vi "Acquisition Message Loop.vi"(8 "error in (no error)":errorcluster, 9 "Data Queue":refnum<queue>, 10 "Data Notifier":refnum<notifier>, 11 "Message Queues":T1) -> (0 "error out":errorcluster)   [LabVIEW 2016, in "Acquisition.lvlib"]
doc: "Message loop for handling messages pertaining to the acquisition of data from the hardware."
uses:
  Acquisition.lvlib
  support/Message Queue/All Message Queues.ctl
  support/Message Queue/Message Cluster.ctl
  Acquisition State.ctl
  Settings/Settings.ctl
  Logging/Logging Configuration.ctl
  Hardware Configuration.ctl
  support/Message Queue/Enqueue Message (Single).vi
  <vilib>/Utility/error.llb/Error Cluster From Error Code.vi
  <vilib>/ErrorRing/Error Ring.xnode
  support/Message Queue/Message Queue.lvlib
  Logging/Logging.lvlib
  Settings/Settings.lvlib
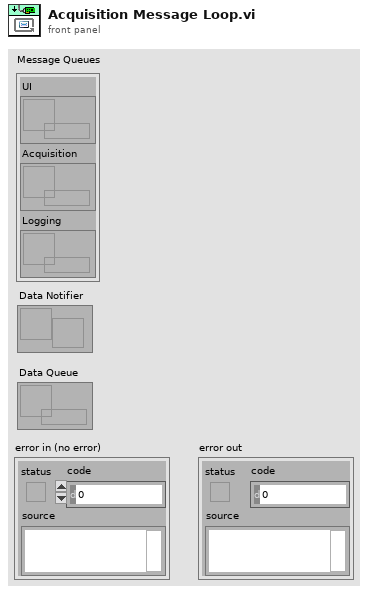
[diagram p1: front panel]
types:
  T1 = typedef "Message Queue.lvlib/All Message Queues.ctl" = cluster{"UI":refnum<queue>, "Acquisition":refnum<queue>, "Logging":refnum<queue>}
  T2 = typedef "Acquisition.lvlib/Acquisition State.ctl" = enum16{"Idle", "Acquiring"}
  T3 = typedef "Settings.lvlib/Settings.ctl" = cluster{"Logging Configuration":T4, "Hardware Config":cluster{"Bautrate":string, "VISA":T5}, "Advance Setting":cluster{"PWM_Step":dbl, "PWM_MIN":dbl, "PWM_MAX":dbl, "DeadZone(mv)":dbl, "SamCycle(ms)":dbl, "Bang-BangTerm":dbl, "ecS":dbl, "ecM":dbl, "ecL":dbl, "eS":dbl, "eM":dbl, "eL":dbl, "Kd F":dbl, "Ki F":dbl, "Kp F":dbl, "Kd":dbl, "Ki":dbl, "Kp":dbl}, "FuzzyMap":cluster{"Table":string[][]}, "ControlMode":cluster{"Control":enum32{"1", "2", "4"}}}
  T4 = typedef "Logging.lvlib/Logging Configuration.ctl" = cluster{"Log File Base Path":path, "save file":bool, "refnum out":refnum<file>}
  T5 = typedef "Acquisition.lvlib/Hardware Configuration.ctl" = refnum<visa-resource-name>
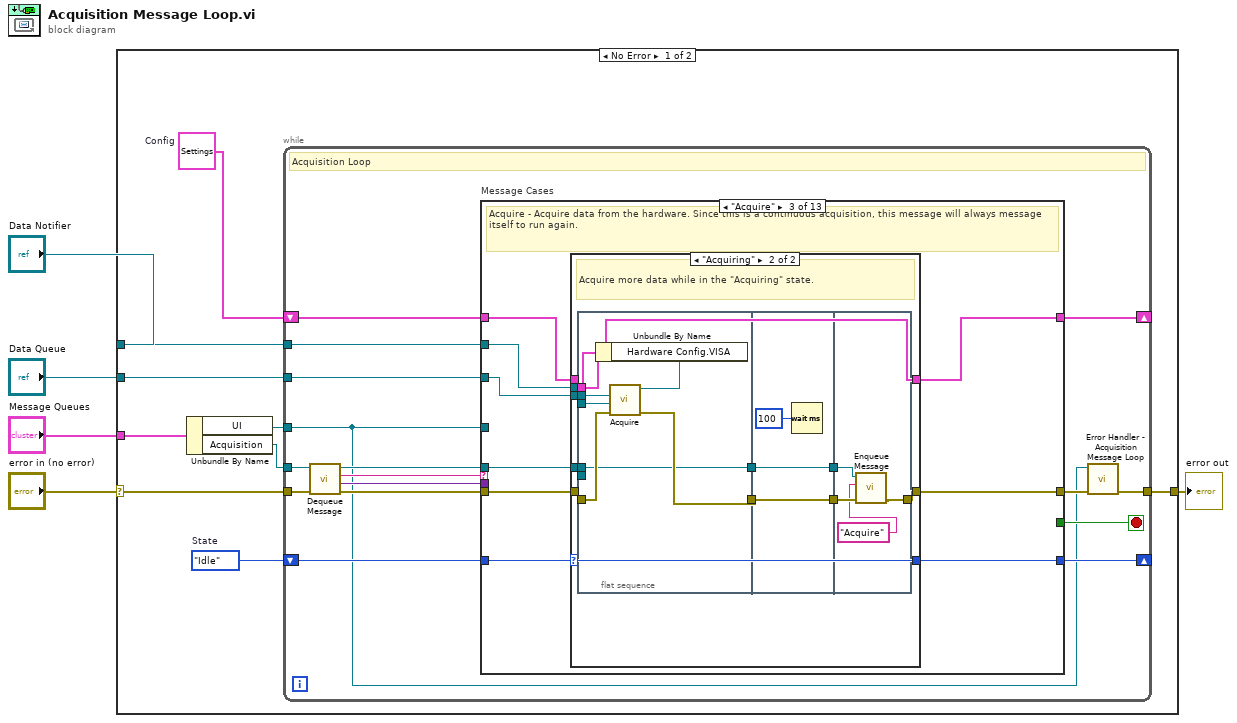
[diagram p0: block diagram]
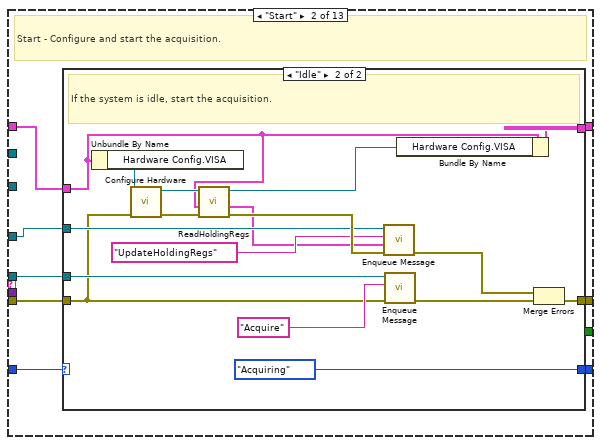
[diagram p3: hidden frame]
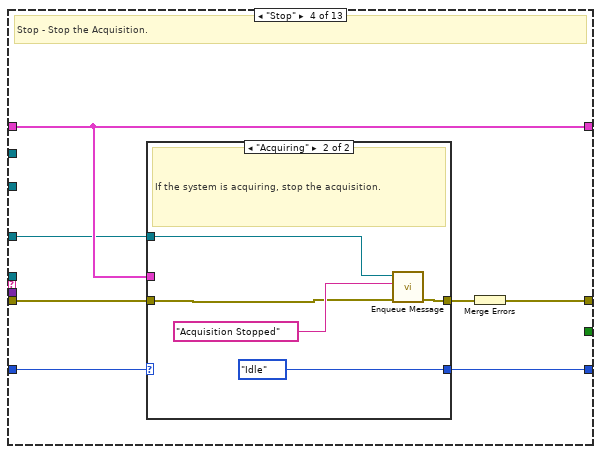
[diagram p6: hidden frame]
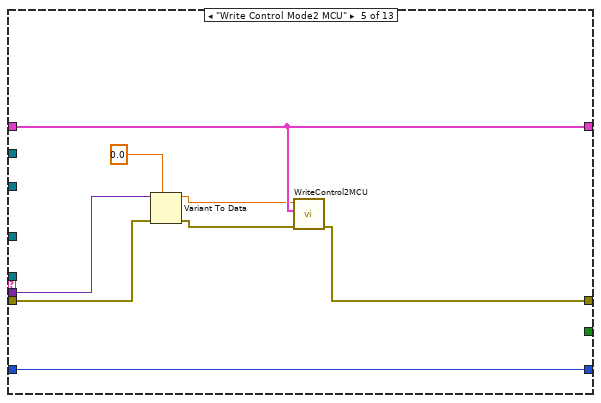
[diagram p8: hidden frame]
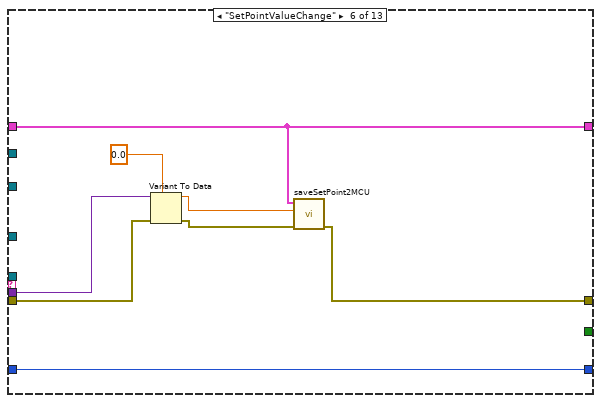
[diagram p9: hidden frame]
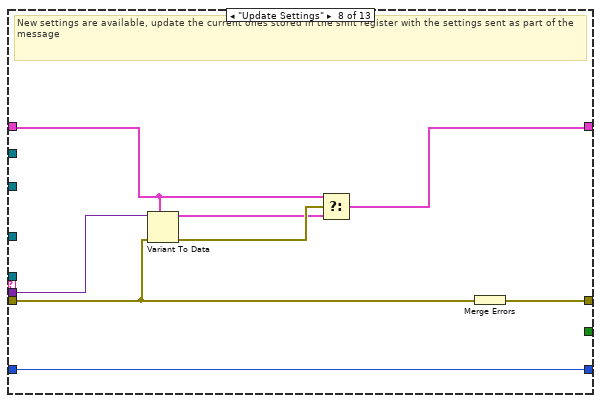
[diagram p11: hidden frame]
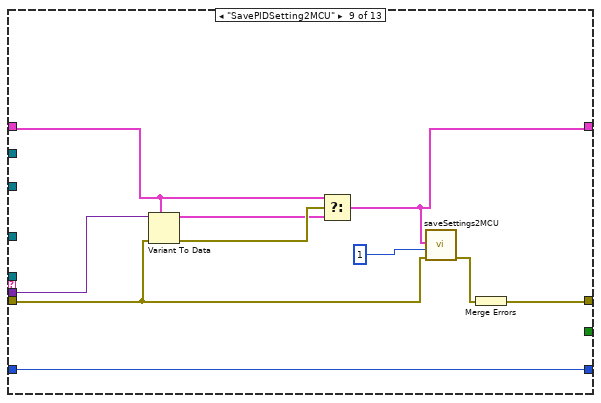
[diagram p12: hidden frame]
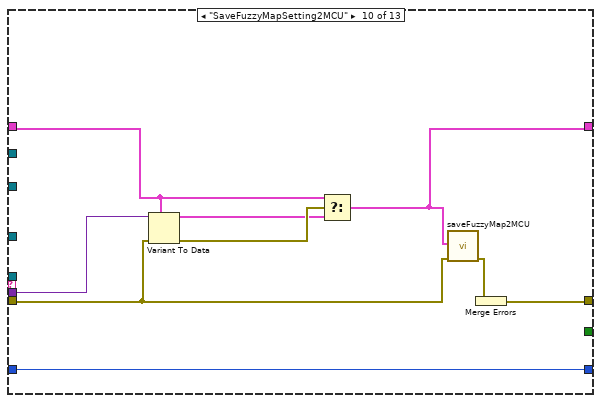
[diagram p13: hidden frame]
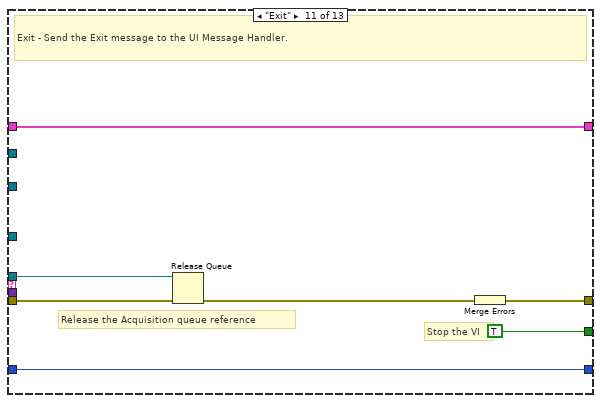
[diagram p14: hidden frame]
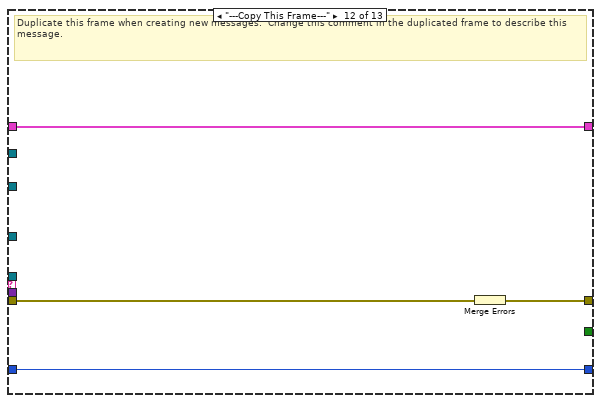
[diagram p15: hidden frame]
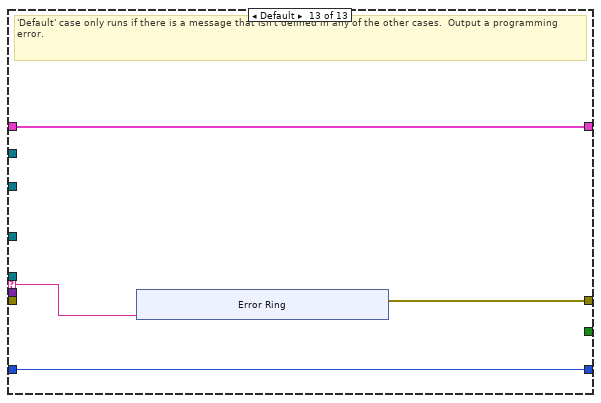
[diagram p16: hidden frame]
diagram:
  n1 = case shown="No Error" "error in (no error)" {
    selector: "error in (no error)" -> [w11 w181]
    tunnel: "Message Queues" -> [w14 _]
    tunnel: [w12 w181] -> w4
    tunnel: "Data Notifier" -> [w9 _]
    tunnel: "Data Queue" -> [w8 _]
    frame No Error {
      w6 = T3 {"Logging Configuration"={"Log File Base Path"=path "", "save file"=FALSE, "refnum out"=refnum}, "Hardware Config"={"Bautrate"="", "VISA"=""}, "Advance Setting"={"PWM_Step"=0.0, "PWM_MIN"=0.0, "PWM_MAX"=0.0, "DeadZone(mv)"=0.0, "SamCycle(ms)"=0.0, "Bang-BangTerm"=0.0, "ecS"=0.0, "ecM"=0.0, "ecL"=0.0, "eS"=0.0, "eM"=0.0, "eL"=0.0, "Kd F"=0.0, "Ki F"=0.0, "Kp F"=0.0, "Kd"=0.0, "Ki"=0.0, "Kp"=0.0}, "FuzzyMap"={"Table"=[]}, "ControlMode"={"Control"=enum."1"}}  # Config
      w7 = Acquisition_State."Idle"  # State
      n2 = Unbundle By Name(w14) -> ("UI"=w10:refnum<queue>, "Acquisition"=w13:refnum<queue>)
      n3 = while {
        tunnel: w13 -> [w23]
        tunnel: w10 -> [w15]
        tunnel: w9 -> [w22]
        tunnel: w8 -> [w21]
        shift-right: [w19] -> _
        shift-left: w7 -> [w20]
        tunnel: w11 -> [w27]
        tunnel: [w18] -> w12
        shift-right: [w29] -> _
        shift-left: w6 -> [w30]
        stop <- w28 stop-if-true
        # "Acquisition Loop"
        n4 = call "Dequeue Message.vi"("error in (no error)"=w27, "Message Queue"=w23) -> ("error out"=w26:errorcluster, "Message Data"=w24:variant, "Message"=w25:string, "dup Message Queue"=w16:refnum<queue>)  [unwired: 6 in]
        n5 = case "Message Cases" shown="\"Acquire\"" w25 {
          selector: w25 -> [_ _ _ _ _ _ _ _ _ _ _ _ w170]
          tunnel: w16 -> [_ w38 w69 _ _ _ _ _ _ _ w160 _ _]
          tunnel: w26 -> [w32 w39 w68 w104 w116 w124 w129 w132 w143 w152 w162 w169 _]
          tunnel: [w32 w41 w70 w105 w118 w126 w129 w139 w144 w154 w164 w167 w171] -> w17
          tunnel: w30 -> [w31 w40 w66 w102 w119 w127 w130 w135 w145 w155 w163 w168 w173]
          tunnel: [w31 w37 w67 w102 w119 w127 w130 w133 w141 w150 w163 w168 w173] -> w29
          tunnel: [_ _ _ _ _ _ _ _ _ _ TRUE _ _] -> w28
          tunnel: w24 -> [_ _ _ _ w117 w125 _ w138 w142 w153 _ _ _]
          tunnel: w15 -> [_ w34 _ w99 _ _ _ _ _ _ _ _ _]
          tunnel: w22 -> [_ _ w65 _ _ _ _ _ _ _ _ _ _]
          tunnel: w21 -> [_ _ w64 _ _ _ _ _ _ _ _ _ _]
          tunnel: w20 -> [w33 w35 w62 w101 w120 w128 w131 w134 w149 w158 w159 w166 w172]
          tunnel: [w33 w36 w63 w100 w120 w128 w131 w134 w149 w158 w159 w166 w172] -> w19
          frame "Initialize" {
            # "Initialize  - Initialize is currently a no-op.  The hardware initialization takes place in the 'Start' message."
          }
          frame "Start" {
            # "Start - Configure and start the acquisition."
            n6 = case shown="\"Idle\"" w35 {
              selector: w35 -> [w42 _]
              tunnel: [w43 w61] -> w41
              tunnel: w40 -> [w44 w45]
              tunnel: w39 -> [w43 w50]
              tunnel: w38 -> [_ w59]
              tunnel: [w44 w56] -> w37
              tunnel: [w42 Acquisition_State."Acquiring" ("Acquisition State")] -> w36
              tunnel: w34 -> [_ w52]
              frame "Acquiring" {
                # "The system is already acquiring. Ignore the \"Start\" message."
              }
              frame "Idle" {
                # "If the system is idle, start the acquisition."
                n7 = Unbundle By Name(w45) -> ("Hardware Config.VISA"=w49:T5)
                n8 = call "Configure Hardware.vi"("error in (no error)"=w50, "Hardware Resources in"=w49) -> ("error out"=w55:errorcluster, "Hardware Resources out"=w48:T5)  [unwired: 8 in]
                n9 = call "ReadHoldingRegs.vi"("error in (no error)"=w55, "Config"=w45, "Hardware Resources in"=w48) -> ("error out"=w54:errorcluster, "output cluster"=w51:T3, "Hardware Resources out"=w47:T5)  [unwired: 6 in]
                n10 = call-poly "Enqueue Message.vi"("error in (no error)"=w54, "Message Data"=w51, "Message"="UpdateHoldingRegs", "Message Queue"=w52) -> ("error out"=w46:errorcluster)  [unwired: 6 in, 1 out]
                n11 = call-poly "Enqueue Message.vi"("error in (no error)"=w50, "Message"="Acquire", "Message Queue"=w59) -> ("error out"=w60:errorcluster)  [unwired: 7 in, 1 out]
                n12 = Bundle By Name(cluster=w45, "Hardware Config.VISA"=w47) -> (w56:T3)
                n13 = Merge Errors(w46, w60) -> (w61:errorcluster)
              }
            }
          }
          frame "Acquire" {
            # "Acquire - Acquire data from the hardware. Since this is a continuous acquisition, this message will always message itself to run again."
            n14 = case shown="\"Acquiring\"" w62 {
              selector: w62 -> [w71 w82]
              tunnel: [w72 w74] -> w70
              tunnel: w69 -> [_ w77]
              tunnel: w68 -> [w72 w81]
              tunnel: [w73 w80] -> w67
              tunnel: w66 -> [w73 w80]
              tunnel: w65 -> [_ w84]
              tunnel: w64 -> [_ w83]
              tunnel: [w71 w82] -> w63
              frame "Idle" {
                # "Ignore \"Acquire\" messages when the acquisition is idle."
              }
              frame "Acquiring" {
                # "Acquire more data while in the \"Acquiring\" state."
                n15 = flat-sequence {
                  tunnel: w77 -> [_]
                  tunnel: w84 -> [w91]
                  tunnel: w83 -> [w90]
                  tunnel: w81 -> [w87]
                  tunnel: w80 -> [w88]
                  tunnel: [w86] -> w79
                  tunnel: w77 -> [w85]
                  tunnel: [w85] -> w76
                  tunnel: w79 -> [w94]
                  tunnel: [w94] -> w78
                  tunnel: w76 -> [w92]
                  tunnel: [w92] -> w75
                  tunnel: w78 -> [w97]
                  tunnel: w75 -> [w98]
                  tunnel: [w96] -> w74
                  frame #0 {
                    n16 = Unbundle By Name(w88) -> ("Hardware Config.VISA"=w89:T5)
                    n17 = call "Acquire.vi"("error in (no error)"=w87, "Data Queue"=w90, "Data Notifier"=w91, "Hardware Resources in"=w89) -> ("error out"=w86:errorcluster)  [unwired: 6 in, 1 out]
                  }
                  frame #1 {
                    n18 = Wait (ms)(milliseconds to wait=u32 100) -> ()  [unwired: 1 out]
                  }
                  frame #2 {
                    n19 = call-poly "Enqueue Message.vi"("error in (no error)"=w97, "Message"="Acquire", "Message Queue"=w98) -> ("error out"=w96:errorcluster)  [unwired: 7 in, 1 out]
                  }
                }
              }
            }
          }
          frame "Stop" {
            # "Stop - Stop the Acquisition."
            n20 = case shown="\"Acquiring\"" w101 {
              selector: w101 -> [w106 _]
              tunnel: w104 -> [w107 w108]
              tunnel: [w107 w111] -> w103
              tunnel: w102 -> [_ _]
              tunnel: [w106 Acquisition_State."Idle" ("State")] -> w100
              tunnel: w99 -> [_ w110]
              frame "Idle" {
                # "The system is already idle. Ignore the \"Stop\" message."
              }
              frame "Acquiring" {
                # "If the system is acquiring, stop the acquisition."
                n21 = call-poly "Enqueue Message.vi"("error in (no error)"=w108, "Message"="Acquisition Stopped", "Message Queue"=w110) -> ("error out"=w111:errorcluster)  [unwired: 7 in, 1 out]
              }
            }
            n22 = Merge Errors(w103) -> (w105:errorcluster)
          }
          frame "Write Control Mode2 MCU" {
            n23 = Variant To Data(error in=w116, type=0.0, Variant=w117) -> (data=w114:dbl, error out=w115:errorcluster)
            n24 = call "WriteControl2MCU.vi"("error in (no error)"=w115, "Config"=w119, "Control Code"=w114) -> ("error out"=w118:errorcluster)  [unwired: 6 in]
          }
          frame "SetPointValueChange" {
            n25 = Variant To Data(error in=w124, type=0.0, Variant=w125) -> (data=w122:dbl, error out=w123:errorcluster)
            n26 = call "saveSetPoint2MCU.vi"("error in (no error)"=w123, "SetPoint"=w122, "Config"=w127) -> ("error out"=w126:errorcluster)  [unwired: 8 in]
          }
          frame "Reset" {
          }
          frame "Update Settings" {
            # "New settings are available, update the current ones stored in the shift register with the settings sent as part of the message"
            n27 = Variant To Data(error in=w132, type=w135, Variant=w138) -> (data=w136:T3, error out=w137:errorcluster)
            n28 = Select(t=w135, s=w137, f=w136) -> (s? t:f=w133:T3)
            n29 = Merge Errors(w132) -> (w139:errorcluster)
          }
          frame "SavePIDSetting2MCU" {
            n30 = Variant To Data(error in=w143, type=w145, Variant=w142) -> (data=w147:T3, error out=w148:errorcluster)
            n31 = Select(t=w145, s=w148, f=w147) -> (s? t:f=w141:T3)
            n32 = call "saveSettings2MCU.vi"("error in (no error)"=w143, "Starting Address"=u16 1, "Config"=w141) -> ("error out"=w146:errorcluster)  [unwired: 6 in]
            n33 = Merge Errors(w146) -> (w144:errorcluster)
          }
          frame "SaveFuzzyMapSetting2MCU" {
            n34 = Variant To Data(error in=w152, type=w155, Variant=w153) -> (data=w156:T3, error out=w157:errorcluster)
            n35 = Select(t=w155, s=w157, f=w156) -> (s? t:f=w150:T3)
            n36 = call "saveFuzzyMap2MCU.vi"("Config"=w150, "error in (no error)"=w152) -> ("error out"=w151:errorcluster)  [unwired: 8 in]
            n37 = Merge Errors(w151) -> (w154:errorcluster)
          }
          frame "Exit" {
            # "Release the Acquisition queue reference"
            # "Stop the VI"
            # "Exit - Send the Exit message to the UI Message Handler."
            n38 = Release Queue(queue=w160, error in (no error)=w162) -> (error out=w161:errorcluster)  [unwired: 1 in, 2 out]
            n39 = Merge Errors(w161) -> (w164:errorcluster)
          }
          frame "---Copy This Frame---" {
            # "Duplicate this frame when creating new messages.  Change this comment in the duplicated frame to describe this message."
            n40 = Merge Errors(w169) -> (w167:errorcluster)
          }
          frame Default {
            # "'Default' case only runs if there is a message that isn't defined in any of the other cases.  Output a programming error."
            n41 = xnode "Error Ring"("parameter 0"=w170) -> ("error out"=w171:errorcluster)
          }
        }
        n42 = call "Error Handler - Acquisition Message Loop.vi"("error in (no error)"=w17, "Message Queue"=w15) -> ("dup error in"=w18:errorcluster)  [unwired: 8 in, 1 out]
      }
    }
    frame Error {
    }
  }
  "error out" <- w4
